vi "FTW-JSON-CodeGen-Image.vi"(0 "State In":T1, 5 "XRef":refnum<vi>) -> (4 "Image":picture)   [LabVIEW 2012, in "FTW-JSON-Deserialize.xnode"]
uses:
  src/JSON/FTW-JSON-Deserialize.xnode
  FTW-JSON-CodeGen-State.ctl
panel:
  # "Inputs"
  # "Outputs"
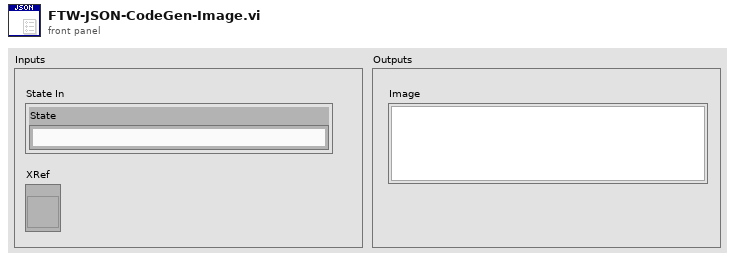
[diagram p1: front panel]
types:
  T1 = typedef "FTW-JSON-Deserialize.xnode/FTW-JSON-CodeGen-State.ctl" = cluster{"State":string}
  T2 = typedef "imagedata.ctl" = cluster{"image type":i32, "image depth":i32, "image":u8[], "mask":u8[], "colors":u32[], "Rectangle":cluster{"left":i16, "top":i16, "right":i16, "bottom":i16}}
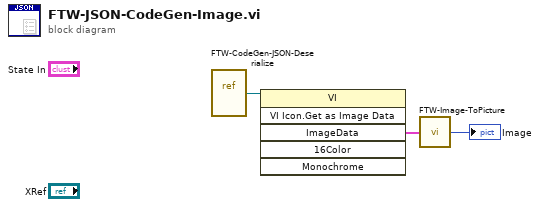
[diagram p0: block diagram]
diagram:
  n1 = vi-ref "FTW-CodeGen-JSON-Deserialize.vi"() -> (w3:refnum<vi>)
  n2 = invoke class="VI" method="VI Icon.Get as Image Data"(reference=w3) -> ("ImageData"=w2:T2)  [unwired: 5 in, 5 out]
  n3 = call "FTW-Image-ToPicture.vi"("Image"=w2) -> ("Picture"=→"Image":picture)
